vi "Find Name and Unit from String.vi"(0 "Input String":string) -> (14 "Units":string, 16 "Signal Name":string)   [LabVIEW 2022 SP3, in "TEXT.lvclass"]
uses:
  TEXT.lvclass
  <vilib>/Utility/error.llb/Trim Whitespace One-Sided.vi
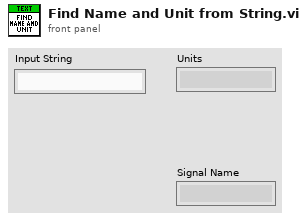
[diagram p1: front panel]
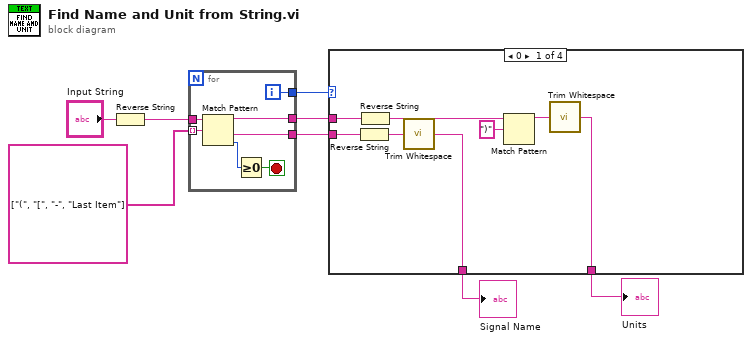
[diagram p0: block diagram]
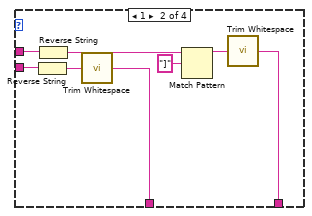
[diagram p2: hidden frame]
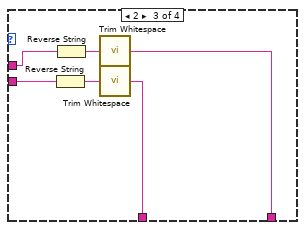
[diagram p3: hidden frame]
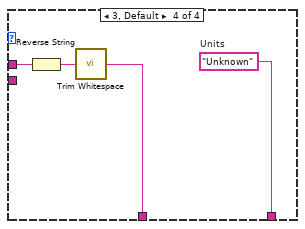
[diagram p4: hidden frame]
diagram:
  n1 = Reverse String(1:"Input String") -> (0:w2:string)
  n2 = for {
    tunnel: w2 -> [w15]
    tunnel: string[] ["(", "[", "-", "Last Item"] -> [w14] mode=indexing
    tunnel: [w11] -> w4
    tunnel: [w10] -> w5
    tunnel: [w9] -> w6
    i -> [w11]
    stop <- w12 stop-if-true
    n3 = Match Pattern(string=w15, regular expression=w14) -> (before substring=w9:string, after substring=w10:string, offset past match=w13:i32)  [unwired: 1 in, 1 out]
    n4 = Greater Or Equal To 0?(x=w13) -> (x >= 0?=w12:bool)
  }
  n5 = case shown="0" w4 {
    tunnel: w5 -> [w22 w26 w37 _]
    tunnel: w6 -> [w21 w27 w36 w38]
    tunnel: [w17 w24 w32 w40] -> w8
    tunnel: [w16 w25 w33 w39] -> w7
    frame 0 {
      n6 = Reverse String(1:w22) -> (0:w23:string)
      n7 = Reverse String(1:w21) -> (0:w20:string)
      n8 = call <vilib>:"Trim Whitespace.vi"("string"=w23) -> ("trimmed string"=w16:string)  [unwired: 1 in]
      n9 = Match Pattern(string=w20, regular expression=")") -> (before substring=w18:string)  [unwired: 1 in, 3 out]
      n10 = call <vilib>:"Trim Whitespace.vi"("string"=w18) -> ("trimmed string"=w17:string)  [unwired: 1 in]
    }
    frame 1 {
      n11 = Reverse String(1:w26) -> (0:w31:string)
      n12 = Reverse String(1:w27) -> (0:w30:string)
      n13 = call <vilib>:"Trim Whitespace.vi"("string"=w31) -> ("trimmed string"=w25:string)  [unwired: 1 in]
      n14 = Match Pattern(string=w30, regular expression="]") -> (before substring=w28:string)  [unwired: 1 in, 3 out]
      n15 = call <vilib>:"Trim Whitespace.vi"("string"=w28) -> ("trimmed string"=w24:string)  [unwired: 1 in]
    }
    frame 2 {
      n16 = Reverse String(1:w37) -> (0:w35:string)
      n17 = Reverse String(1:w36) -> (0:w34:string)
      n18 = call <vilib>:"Trim Whitespace.vi"("string"=w34) -> ("trimmed string"=w32:string)  [unwired: 1 in]
      n19 = call <vilib>:"Trim Whitespace.vi"("string"=w35) -> ("trimmed string"=w33:string)  [unwired: 1 in]
    }
    frame 3, Default {
      w40 = "Unknown"  # Units
      n20 = Reverse String(1:w38) -> (0:w41:string)
      n21 = call <vilib>:"Trim Whitespace.vi"("string"=w41) -> ("trimmed string"=w39:string)  [unwired: 1 in]
    }
  }
  "Units" <- w8
  "Signal Name" <- w7
